vi "fgv_pid_param-var.vi"(7 "cmd":T3=enum."write", 11 "pid-vars_in":T1) -> (3 "pid-var_output":T2 {"deg_agv-center" format="%.1f"; "dis-gap" format="%.1f"; "pid output" format="%.1f"; "deg_agv-lookahead" format="%.1f"; "deg_waypoint" format="%.1f"; "deg_gap" format="%.1f"; "deg_target" format="%.1f"})   [LabVIEW 2019]
uses:
  Ctrl/pid-in-params.ctl
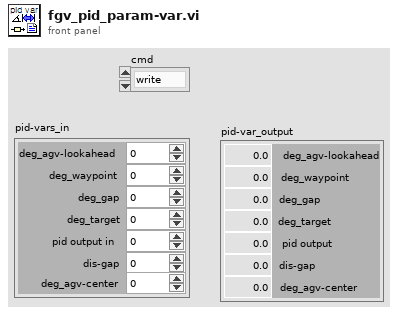
[diagram p1: front panel]
types:
  T1 = cluster{"deg_waypoint":dbl, "deg_agv-lookahead":dbl, "deg_gap":dbl, "deg_target":dbl, "pid output in":dbl, "dis-gap":dbl, "deg_agv-center":dbl}
  T2 = cluster{"deg_agv-lookahead":dbl, "deg_waypoint":dbl, "deg_gap":dbl, "deg_target":dbl, "pid output":dbl, "dis-gap":dbl, "deg_agv-center":dbl}
  T3 = typedef "pid-in-params.ctl" = enum16{"read", "write"}
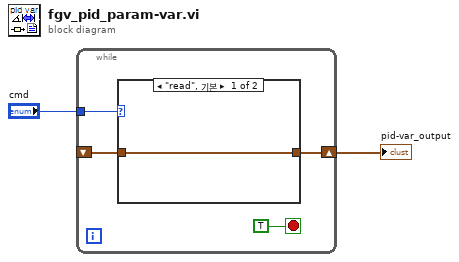
[diagram p0: block diagram]
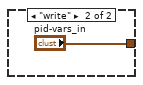
[diagram p2: hidden frame]
diagram:
  n1 = while {
    tunnel: "cmd" -> [w5]
    shift-right: [w4] -> w1
    shift-left: _ -> [w3]
    stop <- TRUE stop-if-true
    n2 = case shown="\"read\", 기본" w5 {
      tunnel: [w7 "pid-vars_in"] -> w4
      tunnel: w3 -> [w7 _]
      frame "read", Default {
      }
      frame "write" {
      }
    }
  }
  "pid-var_output" <- w1
